vi "TagDB-Timestamp.vi"(8 "error in (no error)":errorcluster, 11 "DB Ref":T1) -> (0 "error in (no error) (dup)":errorcluster, 1 "Item Change Timestamp":timestamp, 2 "Global Change Timestamp":timestamp, 3 "DB Ref (dup)":T1)   [LabVIEW 2017, in "TagDB(DEV).lvlib"]
uses:
  TagDB(DEV).lvlib
  Typedef/TagContainer.ctl
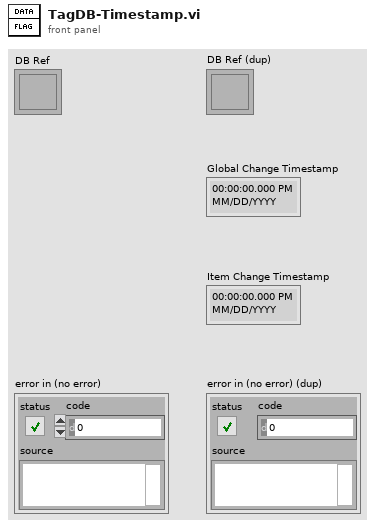
[diagram p1: front panel]
types:
  T1 = typedef "TagDB(DEV).lvlib/TagContainer.ctl" = refnum<k1>
  T2 = typedef "TagContainer.lvlib/tagcontainer-data.ctl" = cluster{"tag-map":variant, "timestamp-map":variant, "namecacher-map":variant, "DataTypeCacher-map":variant, "Tag Adding Lock?":bool, "Global Change Timestamp":timestamp, "Item Change Timestamp":timestamp, "name":string}
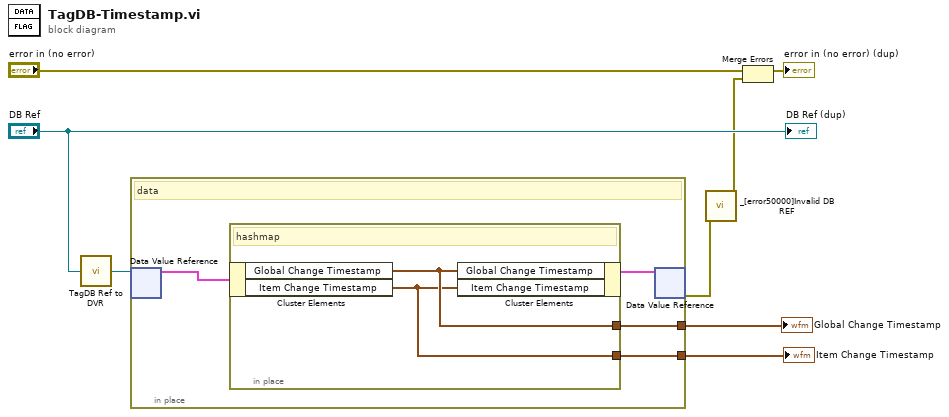
[diagram p0: block diagram]
diagram:
  n1 = call "TagDB Ref to DVR.vi"("TagDB"="DB Ref") -> ("DVR"=w6:refnum<data-value>)  [unwired: 4 in]
  n2 = in-place {
    in-place-border: [w10] -> w1
    in-place-border: [w9] -> w2
    # "data"
    n3 = in-place-dvr #1(w6) -> (w12:T2)  [unwired: 1 out]
    n4 = in-place {
      in-place-border: [w14] -> w10
      in-place-border: [w13] -> w9
      # "hashmap"
      n5 = in-place-cluster #2(w12) -> ("Global Change Timestamp"=w14:timestamp, "Item Change Timestamp"=w13:timestamp)
      n6 = in-place-cluster #2("Global Change Timestamp"=w14, "Item Change Timestamp"=w13) -> (w11:T2)
    }
    n7 = in-place-dvr #1(w11) -> (w5:errorcluster)  [unwired: 1 out]
  }
  "Item Change Timestamp" <- w2
  "Global Change Timestamp" <- w1
  n8 = call "_[error50000]Invalid DB REF.vi"("error in (no error)"=w5) -> ("error out"=w3:errorcluster)  [unwired: 10 in]
  n9 = Merge Errors("error in (no error)", w3) -> (→"error in (no error) (dup)":errorcluster)
  "DB Ref (dup)" <- "DB Ref"
